vi "SetGlobalVariables.vi"   [LabVIEW 2020]
doc: "This VI sets non-robot specific constants and initializes critical global variables."
uses:
  GlobalMiscellaneous.vi
  GlobalDrivebase.vi
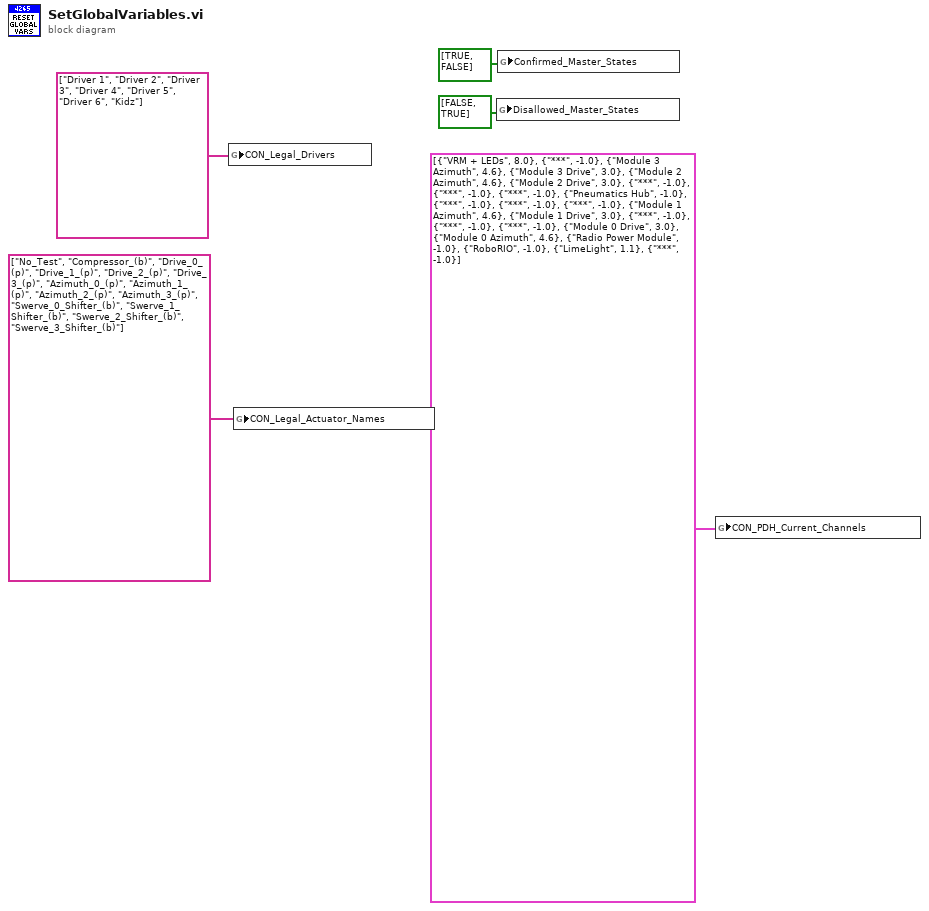
[diagram p0: block diagram]
diagram:
  n1 = global write "GlobalDrivebase.vi" "CON_Legal_Drivers"(string[] ["Driver 1", "Driver 2", "Driver 3", "Driver 4", "Driver 5", "Driver 6", "Kidz"] ("appended array")) -> ()
  n2 = global write "GlobalMiscellaneous.vi" "CON_Legal_Actuator_Names"(string[] ["No_Test", "Compressor_(b)", "Drive_0_(p)", "Drive_1_(p)", "Drive_2_(p)", "Drive_3_(p)", "Azimuth_0_(p)", "Azimuth_1_(p)", "Azimuth_2_(p)", "Azimuth_3_(p)", "Swerve_0_Shifter_(b)", "Swerve_1_Shifter_(b)", "Swerve_2_Shifter_(b)", "Swerve_3_Shifter_(b)"] ("appended array")) -> ()
  n3 = global write "GlobalMiscellaneous.vi" "Disallowed_Master_States"(bool[] [FALSE, TRUE] ("Disallowed_Master_States")) -> ()
  n4 = global write "GlobalMiscellaneous.vi" "Confirmed_Master_States"(bool[] [TRUE, FALSE] ("Disallowed_Master_States")) -> ()
  n5 = global write "GlobalMiscellaneous.vi" "CON_PDH_Current_Channels"(cluster{string, dbl}[] [{"VRM + LEDs", 8.0}, {"***", -1.0}, {"Module 3 Azimuth", 4.6}, {"Module 3 Drive", 3.0}, {"Module 2 Azimuth", 4.6}, {"Module 2 Drive", 3.0}, {"***", -1.0}, {"***", -1.0}, {"***", -1.0}, {"Pneumatics Hub", -1.0}, {"***", -1.0}, {"***", -1.0}, {"***", -1.0}, {"Module 1 Azimuth", 4.6}, {"Module 1 Drive", 3.0}, {"***", -1.0}, {"***", -1.0}, {"***", -1.0}, {"Module 0 Drive", 3.0}, {"Module 0 Azimuth", 4.6}, {"Radio Power Module", -1.0}, {"RoboRIO", -1.0}, {"LimeLight", 1.1}, {"***", -1.0}]) -> ()
